vi "Reorder 2D Array2 (CSG)__ogtk.vi"(8 "reorder (rows)":enum16{"rows", "columns"}(ring), 9 "indices":i32[](array[numeric]), 11 "array":csg[][](array[numeric]) format="%.2f") -> (3 "reordered array":csg[][](array[numeric]) format="%.2f")   [LabVIEW 2016]
doc: "This polymorphic VI reorders a 1D or 2D <B>array</B> of any size based on the indices you specify. For 2D arrays, it reorders by row or by column."
panel:
  # "Reorder 2D Array\n\nThis polymorphic VI reorders a 1D or 2D array of any size based on the indices you specify.  For 2D arrays, it reorders by row or by column.\n\nPlease visit http://www.OpenG.org to learn about the\nOpen Source LabVIEW software movement.\n\nNOTICE -- YOU MUST LEAVE THIS NOTICE IN PLACE.  PER THE TERMS OF THE LICENSE BELOW, YOU MAY SUBLICENSE THIS SOFTWARE \nIN ANY WAY THAT DOES NOT CONFLICT WITH THIS LICENSE.\n\n### BSD License (http://www.opensource.org/licenses/bsd-license.php) Begin ###\n \nCopyright (c) 2002-2007, Jim Kring <jim@jimkring.com>\nCopyright (c) 2002, Cal-Bay Systems, Inc. <info@calbay.com>\nCopyright (c) 2005, MKS Instruments, Inc., author: Doug Femec<doug_femec@mksinst.com>, IM dafemec\n\nAll rights reserved.\n\nRedistribution and use in source and binary forms, with or without modification, are permitted provided that the following conditions are met:\n\n    * Redistributions of source code must retain the above copyright notice, this list of conditions and the following disclaimer.\n    * Redistributions in binary form must reproduce the above copyright notice, this list of conditions and the following disclaimer in the \n       documentation and/or other materials provided with the distribution.\n    * Neither the name of SciWare, James Kring, Inc., nor the names of its contributors may be used to endorse or promote products derived \n       from this software without specific prior written permission.\n\nTHIS SOFTWARE IS PROVIDED BY THE COPYRIGHT HOLDERS AND CONTRIBUTORS \"AS IS\" AND ANY EXPRESS OR IMPLIED WARRANTIES, \nINCLUDING, BUT NOT LIMITED TO, THE IMPLIED WARRANTIES OF MERCHANTABILITY AND FITNESS FOR A PARTICULAR PURPOSE ARE \nDISCLAIMED. IN NO EVENT SHALL THE COPYRIGHT OWNER OR CONTRIBUTORS BE LIABLE FOR ANY DIRECT, INDIRECT, INCIDENTAL,\n SPECIAL, EXEMPLARY, OR CONSEQUENTIAL DAMAGES (INCLUDING, BUT NOT LIMITED TO, PROCUREMENT OF SUBSTITUTE GOODS OR \nSERVICES; LOSS OF USE, DATA, OR PROFITS; OR BUSINESS INTERRUPTION) HOWEVER CAUSED AND ON ANY THEORY OF LIABILITY, \nWHETHER IN CONTRACT, STRICT LIABILITY, OR TORT (INCLUDING NEGLIGENCE OR OTHERWISE) ARISING IN ANY WAY OUT OF THE USE \nOF THIS SOFTWARE, EVEN IF ADVISED OF THE POSSIBILITY OF SUCH DAMAGE.\n\n### BSD License End ###"
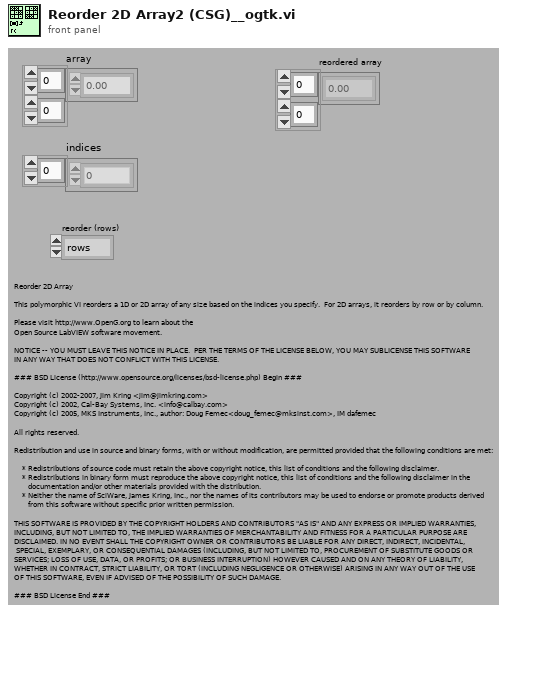
[diagram p1: front panel]
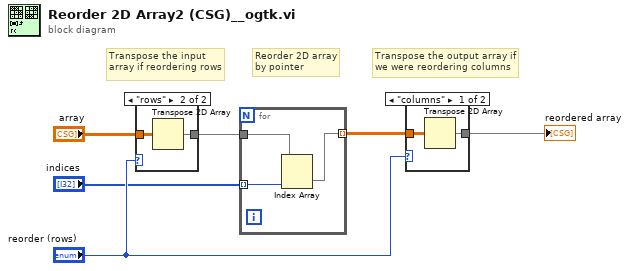
[diagram p0: block diagram]
diagram:
  # "Reorder 2D array by pointer"
  # "Transpose the output array if we were reordering columns"
  # "Transpose the input array if reordering rows"
  n1 = case shown="\"rows\"" "reorder (rows)" {
    tunnel: "array" -> [w7 w9]
    tunnel: [w7 w8] -> w6
    frame "columns" {
      # "Row"
    }
    frame "rows" {
      n2 = Transpose 2D Array(2D array=w9) -> (transposed array=w8:csg[][])
    }
  }
  n3 = for {
    tunnel: w6 -> [w12]
    tunnel: [w11] -> w5 mode=indexing
    tunnel: "indices" -> [w10] mode=indexing
    n4 = Index Array(array=w12, index (col)=w10) -> (element=w11:csg[])  [unwired: 1 in]
  }
  n5 = case shown="\"columns\"" "reorder (rows)" {
    tunnel: w5 -> [w14 w15]
    tunnel: [w13 w15] -> w4
    frame "columns" {
      n6 = Transpose 2D Array(2D array=w14) -> (transposed array=w13:csg[][])
    }
    frame "rows" {
    }
  }
  "reordered array" <- w4
